vi "E7_30.vi"(4 "error in":T15, 7 "Command":T7) -> (0 "error out":T15, 3 "Response":T13)   [LabVIEW 2018]
uses:
  MOKO_LabViewLibrary/MokoLowLevel/MokoLowLovelControl/MLLC_Command.ctl
  MOKO_LabViewLibrary/MokoLowLevel/MokoLowLovelControl/MLLC_Error.ctl
  MOKO_LabViewLibrary/MokoLowLevel/MokoLowLovelControl/MLLC_Mode.ctl
  MOKO_LabViewLibrary/MokoLowLevel/MokoLowLovelControl/MLLC_Response.ctl
  MOKO_LabViewLibrary/MokoLowLevel/MokoLowLovelControl/MLLC_DriverName.ctl
  MOKO_LabViewLibrary/MokoLowLevel/MokoLowLovelControl/MLLC_ResponseInit.ctl
  MOKO_LabViewLibrary/MokoLowLevel/MokoLowLovelControl/MLLC_ErrorCode.ctl
  MOKO_LabViewLibrary/MokoLowLevel/MokoLowLovelControl/MLLC_Request.ctl
  MOKO_LabViewLibrary/MokoLowLevel/MokoLowLovelControl/MLLC_ConnectCluster.ctl
  MOKO_LabViewLibrary/MokoLowLevel/MokoLowLovelControl/MLLC_InterfaceType.ctl
  MOKO_LabViewLibrary/MokoLowLevel/MokoLowLovelControl/MLLC_OpenedSession.ctl
  MOKO_LabViewLibrary/MokoLowLevel/MokoLowLovelControl/MLLC_InterfaceSettings.ctl
  MOKO_LabViewLibrary/MokoLowLevel/MokoLowLovelControl/MLLC_InterfaceKind.ctl
  E7_28/data/E7_28_DATA.ctl
  MOKO_LabViewLibrary/MokoLowLevel/MokoLowLovelControl/MLLC_Rs232Settings.ctl
panel:
  in  "Settings":T9={"Data"={"Connect"={"InterfaceType"=enum."VISA", "OpenedSession"="", "InterfaceSettings"={"Interface"=enum."RS232", "EOS 4 read"=enum."LF (\\n)", "EOS 4 write"=enum."LF (\\n)", "TMO, ms"=10000, "Sett"=variant(cluster{"Baud Rate":u32, "Data Bits":u16, "Parity":u16, "Stop Bits":u16, "Flow Control":u16, "Eho":bool} {"Baud Rate"=75, "Data Bits"=0, "Parity"=0, "Stop Bits"=0, "Flow Control"=0, "Eho"=FALSE})}}, "Cluster"={"flags"="", "freq"=0, "z"=0.0, "f"=0}, "Delay, ms"=100}, "Saved Data"=variant}
  in  "Request":T10="init"
  in  "Error Code":T8=5422
  in  "ResponseInit":T11="Є@E730"
  in  "Driver Name":T12="E7_30"
  in  "Mode":T14=enum."Check"
  # "E7-30"
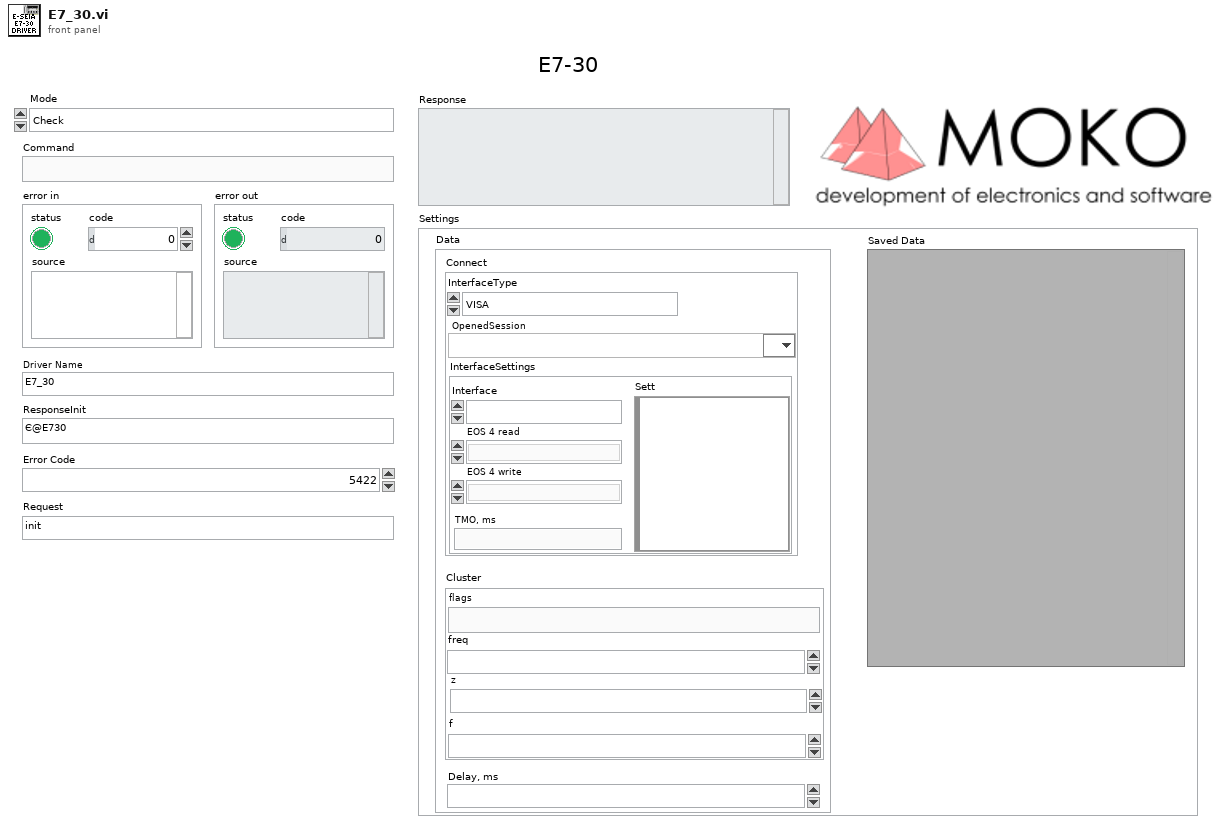
[diagram p1: front panel]
types:
  T1 = typedef "MLLC_ConnectCluster.ctl" = cluster{"InterfaceType":T2, "OpenedSession":T3, "InterfaceSettings":T4}
  T2 = typedef "MLLC_InterfaceType.ctl" = enum16{"VISA", "Prologix USB-GPIB"}
  T3 = typedef "MLLC_OpenedSession.ctl" = refnum<visa-resource-name>
  T4 = typedef "MLLC_InterfaceSettings.ctl" = cluster{"Interface":T5, "EOS 4 read":enum16{"Default (=EOS 4 write)", "CR (\\r)", "LF (\\n)", "None"}, "EOS 4 write":enum16{"CR+LF (\\r\\n)", "CR (\\r)", "LF (\\n)", "None"}, "TMO, ms":i32, "Sett":variant}
  T5 = typedef "MLLC_InterfaceKind.ctl" = enum16{"RS232", "GPIB", "USB", "Ethernet", "another"}
  T6 = typedef "E7_28_DATA.ctl" = cluster{"flags":T7, "freq":T8, "z":dbl, "f":T8}
  T7 = typedef "MLLC_Command.ctl" = string
  T8 = typedef "MLLC_ErrorCode.ctl" = u32
  T9 = cluster{"Data":cluster{"Connect":T1, "Cluster":T6, "Delay, ms":T8}, "Saved Data":variant}
  T10 = typedef "MLLC_Request.ctl" = string
  T11 = typedef "MLLC_ResponseInit.ctl" = string
  T12 = typedef "MLLC_DriverName.ctl" = string
  T13 = typedef "MLLC_Response.ctl" = string
  T14 = typedef "MLLC_Mode.ctl" = enum16{"get", "set", "close", "Init", "Check"}
  T15 = typedef "MLLC_Error.ctl" = errorcluster
  T16 = cluster{"Connect":T1, "Cluster":T6, "Delay, ms":T8}
  T17 = typedef "MLLC_Rs232Settings.ctl" = cluster{"Baud Rate":u32, "Data Bits":u16, "Parity":u16, "Stop Bits":u16, "Flow Control":u16, "Eho":bool, "Address":dbl}
  T18 = typedef "E7_30_DATA.ctl" = cluster{"flags":string, "freq":dbl, "z":dbl, "f":dbl}
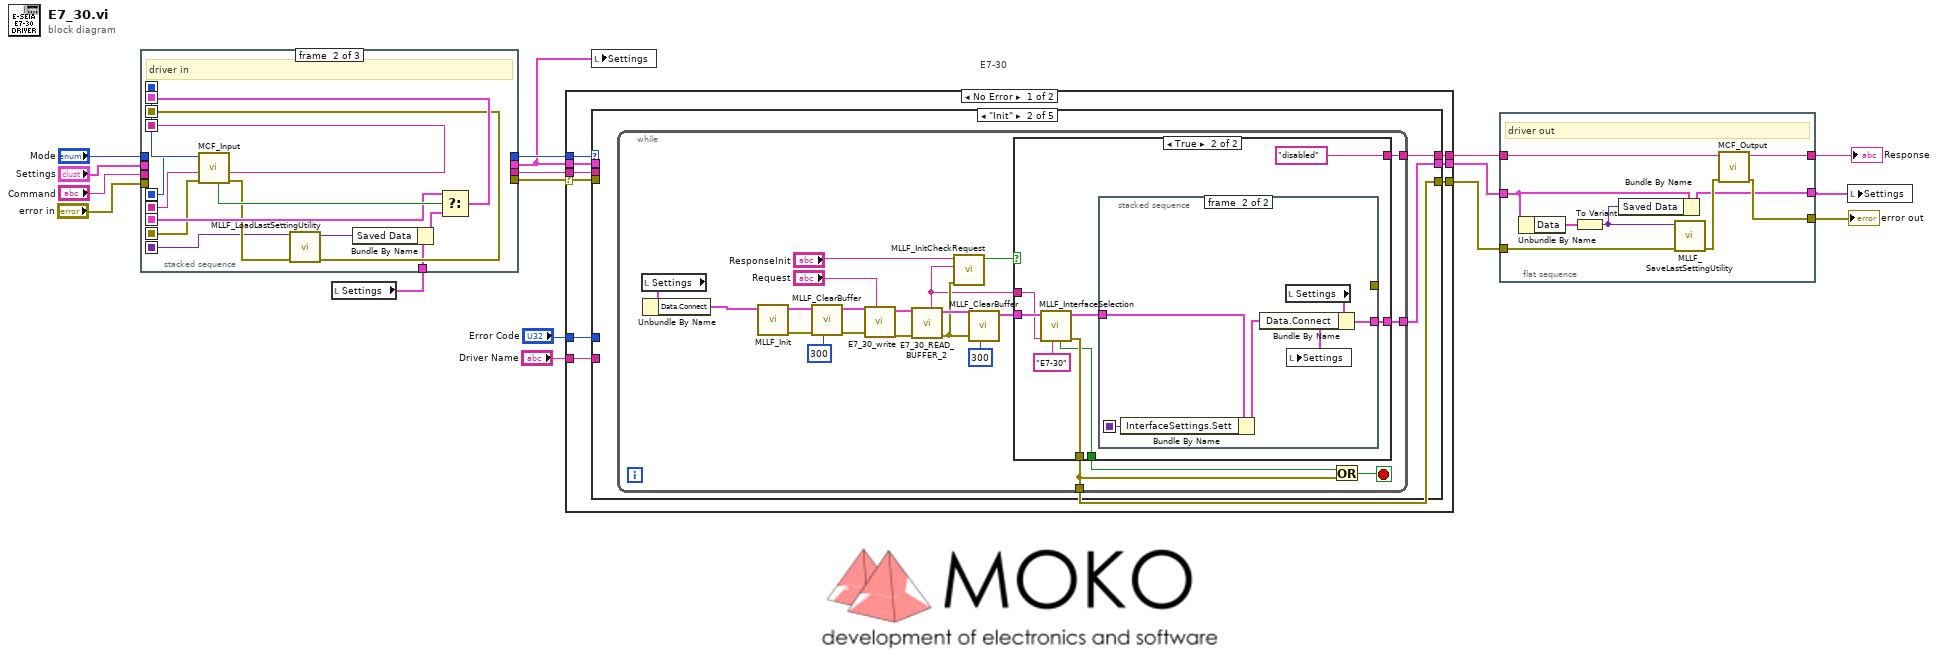
[diagram p0: block diagram]
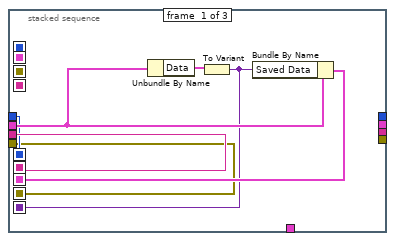
[diagram p2: hidden frame]
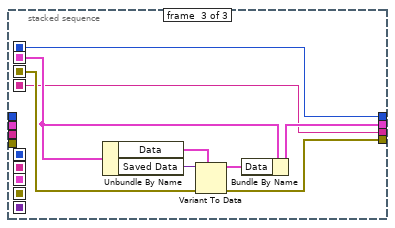
[diagram p3: hidden frame]
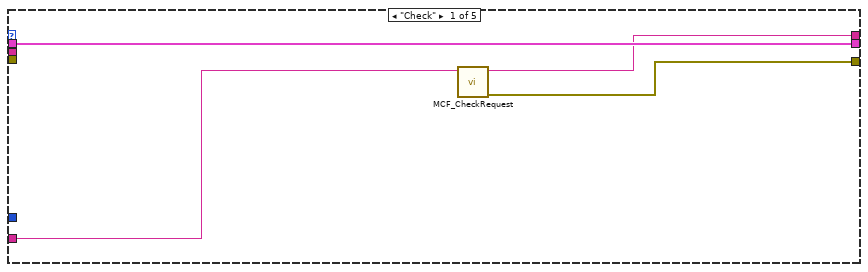
[diagram p4: hidden frame]
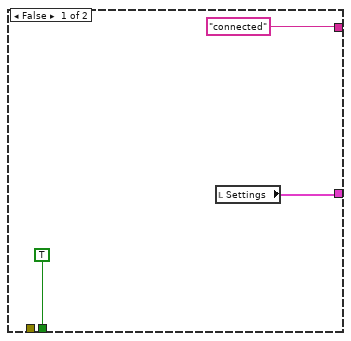
[diagram p5: hidden frame]
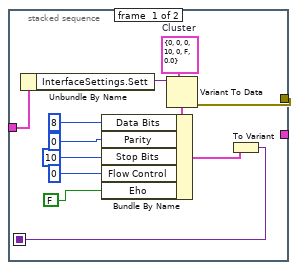
[diagram p6: hidden frame]
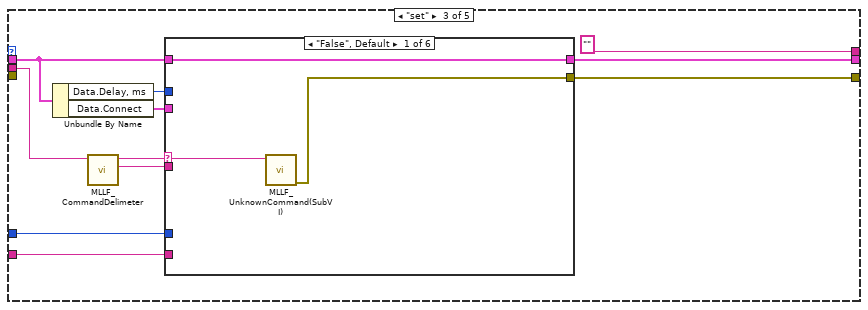
[diagram p7: hidden frame]
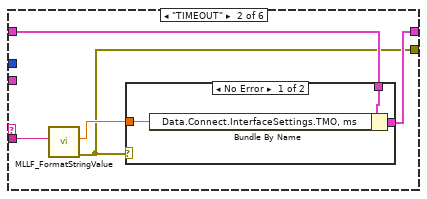
[diagram p8: hidden frame]
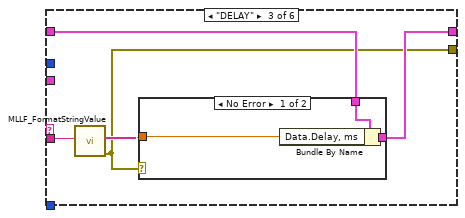
[diagram p10: hidden frame]
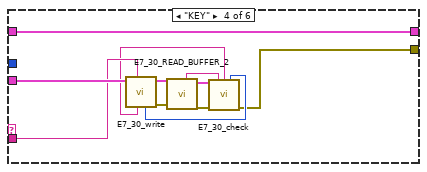
[diagram p12: hidden frame]
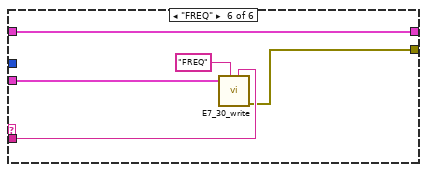
[diagram p14: hidden frame]
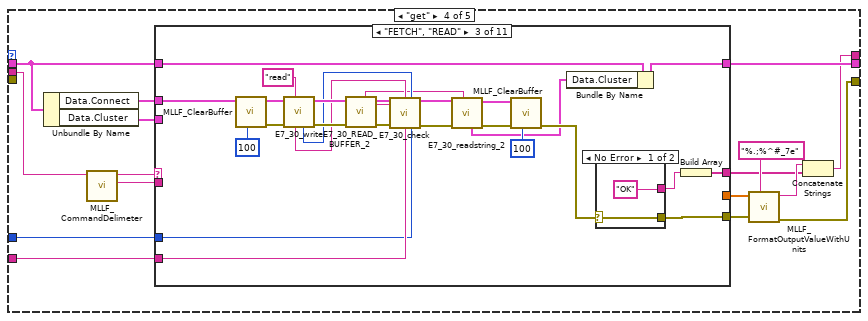
[diagram p15: hidden frame]
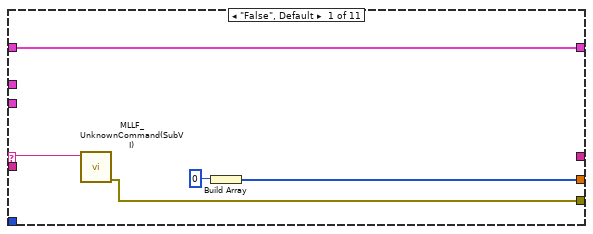
[diagram p16: hidden frame]
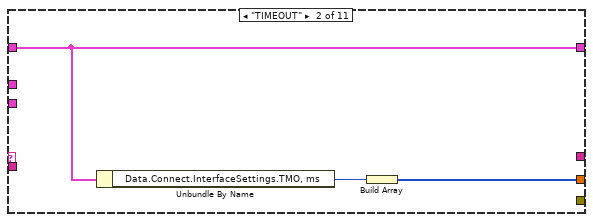
[diagram p17: hidden frame]
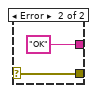
[diagram p18: hidden frame]
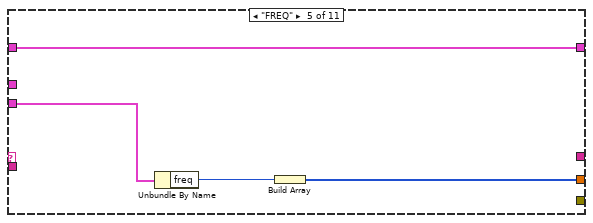
[diagram p20: hidden frame]
diagram:
  # "E7-30"
  n1 = local read "Settings"() -> (w7:T9)
  n2 = stacked-sequence {
    seq-local: [w20 _ _] -> [_ w36 _]
    seq-local: [w19 _ _] -> [_ w37 _]
    seq-local: [w22 _ _] -> [_ w32 _]
    seq-local: [w18 _ _] -> [_ w31 _]
    seq-local: [w21 _ _] -> [_ w27 _]
    seq-local: [_ w28 _] -> [_ _ w44]
    seq-local: [_ w38 _] -> [_ _ w41]
    seq-local: [_ w35 _] -> [_ _ w40]
    seq-local: [_ w34 _] -> [_ _ w45]
    tunnel: "Command" -> [w20 _ _]
    tunnel: "Mode" -> [w19 _ _]
    tunnel: "error in" -> [w18 _ _]
    tunnel: "Settings" -> [w23 _ _]
    tunnel: w7 -> [_ w26 _]
    tunnel: [_ _ w40] -> w9
    tunnel: [_ _ w43] -> w10
    tunnel: [_ _ w42] -> w8
    tunnel: [_ _ w41] -> w11
    frame #0 {
      n3 = Unbundle By Name(w23) -> ("Data"=w24:T16)
      n4 = To Variant(anything=w24) -> (Variant=w21:variant)
      n5 = Bundle By Name(cluster=w23, "Saved Data"=w21) -> (w22:T9)
    }
    frame #1 {
      # "driver in"
      n6 = call "MCF_Input.vi"("Error In"=w31, "Command in"=w36, "Mode in"=w37) -> ("Error Out"=w30:errorcluster, "Command out"=w35:string, "Mode out"=w38:T14, "Boolean"=w33:bool)  [unwired: 5 in]
      n7 = call "MLLF_LoadLastSettingUtility.vi"("Error In"=w30, "Save data in"=w27) -> ("Error Out"=w28:errorcluster, "Save data out"=w25:variant)  [unwired: 8 in]
      n8 = Bundle By Name(cluster=w26, "Saved Data"=w25) -> (w29:T9)
      n9 = Select(t=w32, s=w33, f=w29) -> (s? t:f=w34:T9)
    }
    frame #2 {
      n10 = Unbundle By Name(w45) -> ("Data"=w46:T16, "Saved Data"=w39:variant)
      n11 = Variant To Data(error in=w44, type=w46, Variant=w39) -> (data=w47:T16, error out=w42:errorcluster)
      n12 = Bundle By Name(cluster=w45, "Data"=w47) -> (w43:T9)
    }
  }
  n13 = case shown="No Error" w8 {
    selector: w8 -> [w52 w282]
    tunnel: [w54 w282] -> w4
    tunnel: w11 -> [w56 _]
    tunnel: [w55 "" ("String")] -> w6
    tunnel: w9 -> [w53 _]
    tunnel: w10 -> [w49 w281]
    tunnel: "Error Code" -> [w51 _]
    tunnel: "Driver Name" -> [w50 _]
    tunnel: [w48 w281] -> w5
    frame No Error {
      n14 = case shown="\"Init\"" w56 {
        tunnel: [w59 w63 "" ("String") w164 _] -> w55
        tunnel: [w58 w62 w114 w163 w278] -> w54
        tunnel: w53 -> [_ _ w117 w167 _]
        tunnel: w52 -> [_ _ _ _ _]
        tunnel: w51 -> [_ _ w124 w176 _]
        tunnel: w50 -> [w57 _ w121 w175 _]
        tunnel: w49 -> [w60 _ w123 w178 w277]
        tunnel: [w60 w61 w122 w177 w277] -> w48
        frame "Check" {
          n15 = call "MCF_CheckRequest.vi"("Driver Name"=w57) -> ("Error Out"=w58:errorcluster, "Output String"=w59:string)  [unwired: 9 in]
        }
        frame "Init" {
          n16 = while {
            tunnel: [w83] -> w62
            tunnel: [w66] -> w63
            tunnel: [w65] -> w61
            stop <- w82 stop-if-true
            n17 = local read "Settings"() -> (w85:T9)
            n18 = Unbundle By Name(w85) -> ("Data.Connect"=w84:T1)
            n19 = call "MLLF_Init.vi"("DriverConnect in"=w84) -> ("Error Out"=w77:errorcluster, "DriverConnect out"=w78:T1)  [unwired: 7 in]
            n20 = call "MLLF_ClearBuffer.vi"("Timeout(default = 300 ms)"=u32 300 ("Timeout"), "Error In"=w77, "DriverConnect in"=w78) -> ("Error Out"=w75:errorcluster, "DriverConnect out"=w76:T1)  [unwired: 5 in, 1 out]
            n21 = call "E7_30_write.vi"("Command"="Request", "error in"=w75, "DriverConnect in"=w76) -> ("error out"=w80:T15, "DriverConnect out"=w79:T1)  [unwired: 5 in, 2 out]
            n22 = call "E7_30_READ_BUFFER_2.vi"("error in"=w80, "DriverConnect in"=w79) -> ("error out"=w68:T15, "DriverConnect out"=w72:T1, "String from device out"=w64:string)  [unwired: 7 in]
            n23 = call "MLLF_InitCheckRequest.vi"("error in (no error)"=w68, "Answer"=w64, "Response Init"="ResponseInit") -> ("Design"=w67:bool)  [unwired: 5 in, 3 out]
            n24 = call "MLLF_ClearBuffer.vi"("Timeout(default = 300 ms)"=u32 300 ("Timeout"), "Error In"=w68, "DriverConnect in"=w72) -> ("DriverConnect out"=w71:T1)  [unwired: 5 in, 2 out]
            n25 = case shown="True" w67 {
              tunnel: [_ w94] -> w83
              tunnel: [TRUE w90] -> w81
              tunnel: w71 -> [_ w96]
              tunnel: ["connected" "disabled"] -> w66
              tunnel: [w86 w91] -> w65
              tunnel: w64 -> [_ w89]
              frame False {
                n26 = local read "Settings"() -> (w86:T9)
              }
              frame True {
                n27 = call "MLLF_InterfaceSelection.vi"("Driver Name"="E7-30" ("String"), "Answer:"=w89, "DriverConnect in"=w96) -> ("error out"=w94:T15, "DriverConnect out"=w95:T1, "stop init?"=w90:bool)  [unwired: 4 in, 2 out]
                n28 = stacked-sequence {
                  seq-local: [w99 _] -> [_ w112]
                  tunnel: w95 -> [w97 w110]
                  tunnel: [w106 _] -> _
                  tunnel: [_ w111] -> w91
                  frame #0 {
                    w107 = T17 {"Baud Rate"=0, "Data Bits"=0, "Parity"=0, "Stop Bits"=10, "Flow Control"=0, "Eho"=FALSE, "Address"=0.0}  # Cluster
                    n29 = Unbundle By Name(w97) -> ("InterfaceSettings.Sett"=w108:variant)
                    n30 = Variant To Data(type=w107, Variant=w108) -> (data=w105:T17, error out=w106:errorcluster)  [unwired: 1 in]
                    n31 = Bundle By Name(cluster=w105, "Data Bits"=u16 8 ("Serial Settings:Data Bits"), "Parity"=u16 0 ("Serial Settings:Parity"), "Stop Bits"=u16 10 ("Serial Settings:Stop Bits"), "Flow Control"=u16 0 ("Serial Settings:Flow Control"), "Eho"=FALSE) -> (w100:T17)
                    n32 = To Variant(anything=w100) -> (Variant=w99:variant)
                  }
                  frame #1 {
                    n33 = Bundle By Name(cluster=w110, "InterfaceSettings.Sett"=w112) -> (w109:T1)
                    n34 = local read "Settings"() -> (w113:T9)
                    n35 = Bundle By Name(cluster=w113, "Data.Connect"=w109) -> (w111:T9)
                    n36 = local write "Settings"(w111) -> ()
                  }
                }
              }
            }
            n37 = Or(x=w81, y=w83) -> (x .or. y?=w82:bool)
          }
        }
        frame "set" {
          n38 = Unbundle By Name(w123) -> ("Data.Delay, ms"=w118:T8, "Data.Connect"=w119:T1)
          n39 = call "MLLF_CommandDelimeter.vi"("command with param"=w117) -> ("param 1"=w115:string, "command"=w116:string)  [unwired: 6 in, 3 out]
          n40 = case shown="\"False\", Default" w116 {
            selector: w116 -> [w126 _ _ _ _ _]
            tunnel: w115 -> [_ w130 w139 w154 _ w159]
            tunnel: [w125 w128 w137 w146 _ w158] -> w114
            tunnel: w124 -> [_ _ _ _ _ _]
            tunnel: w123 -> [w127 w131 w140 w156 w157 w162]
            tunnel: [w127 w132 w141 w156 w157 w162] -> w122
            tunnel: w119 -> [_ _ _ w155 _ w161]
            tunnel: w121 -> [_ _ _ _ _ _]
            tunnel: w118 -> [_ _ _ _ _ _]
            frame "False", Default {
              n41 = call "MLLF_UnknownCommand(SubVI).vi"("Unknown command"=w126) -> ("error out"=w125:errorcluster)  [unwired: 10 in]
            }
            frame "TIMEOUT" {
              n42 = call "MLLF_FormatStringValue.vi"("String Value"=w130) -> ("error out"=w128:T15, "number"=w129:dbl)  [unwired: 8 in, 1 out]
              n43 = case shown="No Error" w128 {
                tunnel: [w135 w136] -> w132
                tunnel: w131 -> [w134 w136]
                tunnel: w129 -> [w133 _]
                frame No Error {
                  n44 = Bundle By Name(cluster=w134, "Data.Connect.InterfaceSettings.TMO, ms"=w133) -> (w135:T9)
                }
                frame Error {
                }
              }
            }
            frame "DELAY" {
              n45 = call "MLLF_FormatStringValue.vi"("String Value"=w139) -> ("error out"=w137:T15, "number"=w138:dbl)  [unwired: 8 in, 1 out]
              n46 = case shown="No Error" w137 {
                tunnel: [w144 w145] -> w141
                tunnel: w140 -> [w143 w145]
                tunnel: w138 -> [w142 _]
                frame No Error {
                  n47 = Bundle By Name(cluster=w143, "Data.Delay, ms"=w142) -> (w144:T9)
                }
                frame Error {
                }
              }
            }
            frame "KEY" {
              n48 = call "E7_30_write.vi"("Command"=w154, "DriverConnect in"=w155) -> ("error out"=w150:T15, "DriverConnect out"=w151:T1, "command HEX out"=w148:T8, "command string out"=w149:T7)  [unwired: 6 in]
              n49 = call "E7_30_READ_BUFFER_2.vi"("error in"=w150, "DriverConnect in"=w151) -> ("error out"=w152:T15, "DriverConnect out"=w153:T1, "String from device out"=w147:string)  [unwired: 7 in]
              n50 = call "E7_30_check.vi"("DriverConnect in"=w153, "String in"=w147, "command string in"=w149, "command HEX in"=w148, "error in"=w152) -> ("error out"=w146:T15)  [unwired: 9 in, 1 out]
            }
            frame "---------------------------------------------------------------------------------------" {
            }
            frame "FREQ" {
              n51 = call "E7_30_write.vi"("VALUE"=w159, "Command"="FREQ", "DriverConnect in"=w161) -> ("error out"=w158:T15)  [unwired: 5 in, 3 out]
            }
          }
        }
        frame "get" {
          n52 = Unbundle By Name(w178) -> ("Data.Connect"=w171:T1, "Data.Cluster"=w168:T6)
          n53 = call "MLLF_CommandDelimeter.vi"("command with param"=w167) -> ("param 1"=w165:string, "command"=w166:string)  [unwired: 6 in, 3 out]
          n54 = case shown="\"FETCH\", \"READ\"" w166 {
            selector: w166 -> [w180 _ _ _ _ _ _ _ _ _ _]
            tunnel: w165 -> [_ _ _ _ _ _ _ _ _ _ _]
            tunnel: [w179 _ w196 _ _ _ _ _ _ _ _] -> w173
            tunnel: w176 -> [_ _ w201 _ _ _ _ _ _ _ _]
            tunnel: [w183 w186 w188 w217 w218 w231 w232 w236 w245 w268 w271] -> w177
            tunnel: [w181 w184 _ _ w219 w225 w233 w237 w247 w258 w272] -> w172
            tunnel: w171 -> [_ _ w206 _ _ _ _ _ _ _ _]
            tunnel: w175 -> [_ _ w202 _ _ _ _ _ _ _ _]
            tunnel: [_ _ w197 _ _ _ _ _ _ _ _] -> w169
            tunnel: w168 -> [_ _ _ _ w221 w230 w235 w239 w251 w259 w274]
            tunnel: w178 -> [w183 w186 w189 w217 w218 w231 w232 w236 w245 w268 w271]
            frame "False", Default {
              n55 = call "MLLF_UnknownCommand(SubVI).vi"("Unknown command"=w180) -> ("error out"=w179:errorcluster)  [unwired: 10 in]
              n56 = Build Array(0 ("TimeOut")) -> (w181:i32[])
            }
            frame "TIMEOUT" {
              n57 = Unbundle By Name(w186) -> ("Data.Connect.InterfaceSettings.TMO, ms"=w185:i32)
              n58 = Build Array(w185) -> (w184:i32[])
            }
            frame "FETCH", "READ" {
              n59 = call "MLLF_ClearBuffer.vi"("Timeout(default = 300 ms)"=u32 100 ("Timeout"), "DriverConnect in"=w206) -> ("Error Out"=w209:errorcluster, "DriverConnect out"=w210:T1)  [unwired: 6 in, 1 out]
              n60 = call "E7_30_write.vi"("Command"="read", "error in"=w209, "DriverConnect in"=w210) -> ("error out"=w212:T15, "DriverConnect out"=w211:T1, "command HEX out"=w199:T8, "command string out"=w200:T7)  [unwired: 5 in]
              n61 = call "E7_30_READ_BUFFER_2.vi"("error in"=w212, "DriverConnect in"=w211) -> ("error out"=w203:T15, "DriverConnect out"=w204:T1, "String from device out"=w193:string)  [unwired: 7 in]
              n62 = call "E7_30_check.vi"("DriverConnect in"=w204, "String in"=w193, "command string in"=w200, "command HEX in"=w199, "error in"=w203, "Driver Name"=w202, "Error Code"=w201) -> ("DriverConnect out"=w195:T1, "error out"=w194:T15)  [unwired: 7 in]
              n63 = call "E7_30_readstring_2.vi"("data string"=w193, "error in"=w194, "DriverConnect in"=w195) -> ("error out"=w191:T15, "DriverConnect out"=w192:T1, "Cluster"=w187:T18)  [unwired: 6 in]
              n64 = call "MLLF_ClearBuffer.vi"("Timeout(default = 300 ms)"=u32 100 ("Timeout"), "Error In"=w191, "DriverConnect in"=w192) -> ("Error Out"=w190:errorcluster)  [unwired: 5 in, 2 out]
              n65 = Bundle By Name(cluster=w189, "Data.Cluster"=w187) -> (w188:T9)
              n66 = case shown="No Error" w190 {
                selector: w190 -> [w214 w215]
                tunnel: [w214 w215] -> w196
                tunnel: ["OK" "OK"] -> w198
                frame No Error {
                }
                frame Error {
                }
              }
              n67 = Build Array(w198) -> (w197:string[])
            }
            frame "---------------------------------------------------------" {
            }
            frame "FREQ" {
              n68 = Unbundle By Name(w221) -> ("freq"=w220:T8)
              n69 = Build Array(w220) -> (w219:T8[])
            }
            frame "R", "Rs" {
              n70 = Unbundle By Name(w230) -> ("f"=w223:T8)
              n71 = Unbundle By Name(w230) -> ("z"=w229:dbl)
              n72 = Divide(x=w223, y=57.2958) -> (x/y=w222:dbl)
              n73 = Absolute Value(x=w229) -> (abs(x)=w228:dbl)
              n74 = Cosine(x=w222) -> (cos(x)=w227:dbl)
              n75 = Multiply(x=w228, y=w227) -> (x*y=w226:dbl)
              n76 = Build Array(w226) -> (w225:dbl[])
            }
            frame "Z" {
              # "Модуль комплексного сопротивления, Z"
              n77 = Unbundle By Name(w235) -> ("z"=w234:dbl)
              n78 = Build Array(w234) -> (w233:dbl[])
            }
            frame "F" {
              # "Фазовый угол"
              n79 = Unbundle By Name(w239) -> ("f"=w238:T8)
              n80 = Build Array(w238) -> (w237:T8[])
            }
            frame "C" {
              # "Емкость С, Ф"
              n81 = Unbundle By Name(w251) -> ("freq"=w250:T8)
              n82 = Unbundle By Name(w251) -> ("z"=w254:dbl)
              n83 = Unbundle By Name(w251) -> ("f"=w241:T8)
              n84 = Divide(x=w241, y=57.2958) -> (x/y=w242:dbl)
              n85 = Sine(x=w242) -> (sin(x)=w253:dbl)
              n86 = Multiply(x=w254, y=w253) -> (x*y=w252:dbl)
              n87 = Multiply(x=w250, y=6.283185307179586) -> (x*y=w248:dbl)
              n88 = Multiply(x=w252, y=w248) -> (x*y=w246:dbl)
              n89 = Reciprocal(x=w246) -> (1/x=w244:dbl)
              n90 = Absolute Value(x=w244) -> (abs(x)=w243:dbl)
              n91 = Build Array(w243) -> (w247:dbl[])
            }
            frame "L" {
              # "?? неправильно считает\nнужно обратиться к разработчику"
              n92 = Unbundle By Name(w259) -> ("freq"=w262:T8)
              n93 = Unbundle By Name(w259) -> ("z"=w256:dbl)
              n94 = Unbundle By Name(w259) -> ("f"=w266:T8)
              n95 = Absolute Value(x=w256) -> (abs(x)=w255:dbl)
              n96 = Divide(x=w266, y=57.2958) -> (x/y=w265:dbl)
              n97 = Sine(x=w265) -> (sin(x)=w260:dbl)
              n98 = Multiply(x=w255, y=w260) -> (x*y=w261:dbl)
              n99 = Multiply(x=w262, y=6.283185307179586) -> (x*y=w264:dbl)
              n100 = Multiply(x=w261, y=w264) -> (x*y=w257:dbl)
              n101 = Build Array(w257) -> (w258:dbl[])
            }
            frame "D" {
              # "Фактор потерь, D"
              n102 = Unbundle By Name(w274) -> ("f"=w276:T8)
              n103 = Divide(x=w276, y=57.2958) -> (x/y=w273:dbl)
              n104 = Tangent(1:w273) -> (0:w270:dbl)
              n105 = Absolute Value(x=w270) -> (abs(x)=w269:dbl)
              n106 = Build Array(w269) -> (w272:dbl[])
            }
          }
          n107 = call "MLLF_FormatOutputValueWithUnits.vi"("Format"="%.;%^#_7e" ("format string"), "error in"=w173, "ValuesIn"=w172) -> ("error out"=w163:T15, "Result string"=w174:T7)  [unwired: 7 in]
          n108 = Concatenate Strings(w174, w169) -> (w164:string)
        }
        frame "close" {
          n109 = Unbundle By Name(w277) -> ("Data.Connect.OpenedSession"=w279:T3)
          n110 = VISA Close(VISA resource name=w279) -> (error out=w278:errorcluster)  [unwired: 1 in]
        }
      }
    }
    frame Error {
    }
  }
  n111 = local write "Settings"(w10) -> ()
  n112 = flat-sequence {
    tunnel: [w291] -> w3
    tunnel: [w290] -> w1
    tunnel: w6 -> [w289]
    tunnel: w4 -> [w288]
    tunnel: w5 -> [w284]
    tunnel: [w286] -> w2
    frame #0 {
      # "driver out"
      n113 = Unbundle By Name(w284) -> ("Data"=w283:T16)
      n114 = To Variant(anything=w283) -> (Variant=w285:variant)
      n115 = Bundle By Name(cluster=w284, "Saved Data"=w285) -> (w286:T9)
      n116 = call "MLLF_SaveLastSettingUtility.vi"("error in"=w288, "Saved Data"=w285) -> ("error out"=w287:T15)  [unwired: 8 in, 1 out]
      n117 = call "MCF_Output.vi"("Error In"=w287, "Input"=w289) -> ("Error Out"=w290:errorcluster, "Output"=w291:string)  [unwired: 8 in]
    }
  }
  n118 = local write "Settings"(w2) -> ()
  "error out" <- w1
  "Response" <- w3
